vi "Get number of channels from digitizer correction file.vi"(11 "Correction file path":path=path "D:/martin/TWM - github/data/corrections/transducers/dummy.vd/dummy.info") -> (3 "Number of channels":u32)   [LabVIEW 2020]
doc: "Reads a digitizer correction file (info format, TWM structure) and finds out the number of channels this correction files covers."
uses:
  TWM - github/lvprog/octave/infolib/Get 1D String.vi
  TWM - github/lvprog/octave/infolib/infolib.lvlib
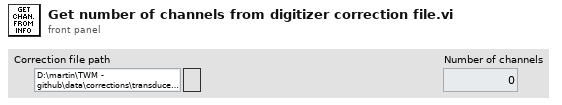
[diagram p1: front panel]
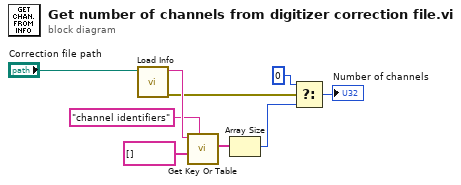
[diagram p0: block diagram]
diagram:
  n1 = call "Load Info.vi"("filename"="Correction file path") -> ("error out"=w4:errorcluster, "info data"=w8:string)  [unwired: 9 in]
  n2 = call-poly "Get Key Or Table.vi"("key description"="channel identifiers", "string"=string[] [], "info data"=w8) -> ("value"=w5:string[])  [unwired: 5 in, 3 out]
  n3 = Array Size(array=w5) -> (size(s)=w3:i32)
  n4 = Select(t=0 ("f"), s=w4, f=w3) -> (s? t:f=→"Number of channels":i32)
